vi "Get Sequences Information for UI.vi"(11 "filtered engines":T1[](array[typedef])) -> (0 "error out":errorcluster, 1 "Steps":string[][](array[string]), 2 "Sequences":string[](array[string]))   [LabVIEW 2015, in "Sequencer Module tests.lvlib"]
uses:
  Sequencer Module tests.lvlib
  <vilib>/NI/DCAF/Tag Editor Core/Framework Configuration Classes/platypus configuration/engines cluster.ctl
  <vilib>/NI/Module Execution Interface/Engine Configuration/engine configuration.lvclass
  <vilib>/NI/Tag Bus Module Framework/module configuration/TBM module configuration.lvclass
  module/configuration/Sequencer Module configuration.lvclass
  module/configuration/Sequencer Module configuration.lvclass/Sequencer Module configuration.ctl
  module/configuration/Read Lines.vi
  classes/Sequence/Config/Sequence Config.lvclass
  classes/Step/Config/Step Config.lvclass
  <vilib>/NI/DCAF/Tag Editor Core/Framework Configuration Classes/platypus configuration/PLConfigurationSerializer.lvlib
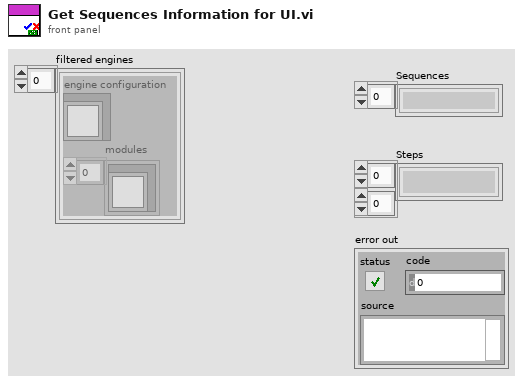
[diagram p1: front panel]
types:
  T1 = typedef "PLConfigurationSerializer.lvlib/engines cluster.ctl" = cluster{"engine configuration":refnum<class "engine configuration.lvclass">, "modules":refnum<class "TBM module configuration.lvclass">[]}
  T2 = typedef "Sequencer Module configuration.lvclass/Line.ctl" = cluster{"Sequence":refnum<class "Sequence Config.lvclass">}
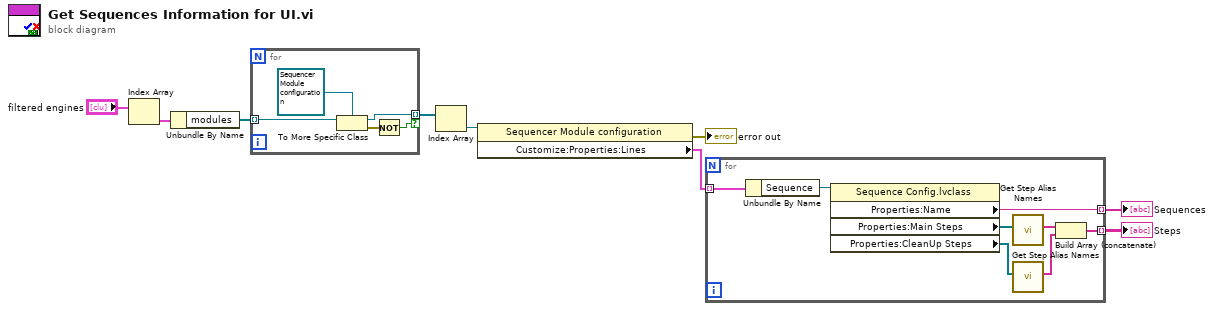
[diagram p0: block diagram]
diagram:
  n1 = Index Array(array="filtered engines") -> (element=w7:T1)  [unwired: 1 in]
  n2 = Unbundle By Name(w7) -> ("modules"=w8:refnum<class "TBM module configuration.lvclass">[])
  n3 = for {
    tunnel: w8 -> [w14] mode=indexing
    tunnel: [w11] -> w9 mode=indexing if=w10
    n4 = To More Specific Class(target class=refnum<class "Sequencer Module configuration.lvclass"> refnum ("Sequencer Module configuration"), reference=w14) -> (specific class reference=w11:refnum<class "Sequencer Module configuration.lvclass">, error out=w12:errorcluster)  [unwired: 1 in]
    n5 = Not(x=w12) -> (.not. x?=w10:bool)
  }
  n6 = Index Array(array=w9) -> (element=w2:refnum<class "Sequencer Module configuration.lvclass">)  [unwired: 1 in]
  n7 = property class="Sequencer Module configuration"(reference=w2) -> (error out=→"error out":errorcluster, "Customize:Properties:Lines"=w3:T2[])  [unwired: 1 in, 1 out]
  n8 = for {
    tunnel: w3 -> [w22] mode=indexing
    tunnel: [w18] -> w4 mode=indexing
    tunnel: [w15] -> w5 mode=indexing
    n9 = Unbundle By Name(w22) -> ("Sequence"=w21:refnum<class "Sequence Config.lvclass">)
    n10 = property class="Sequence Config.lvclass"(reference=w21) -> ("Properties:Name"=w18:string, "Properties:Main Steps"=w20:refnum<class "Step Config.lvclass">[], "Properties:CleanUp Steps "=w19:refnum<class "Step Config.lvclass">[])  [unwired: 1 in, 2 out]
    n11 = call "Get Step Alias Names.vi"("Properties:Main Steps"=w20) -> ("Steps Alias"=w17:string[])  [unwired: 10 in]
    n12 = call "Get Step Alias Names.vi"("Properties:Main Steps"=w19) -> ("Steps Alias"=w16:string[])  [unwired: 10 in]
    n13 = Build Array (concatenate)(w17, w16) -> (w15:string[])
  }
  "Steps" <- w5
  "Sequences" <- w4
